vi "(SubVI)Serial_FGV.vi"(5 "Serial Settings (for init)":T2={"baud rate"=19200, "data bits"=8, "parity"=enum."None", "stop bits"=10, "flow control"=0} {"flow control" items=["None"=0, "XON/XOFF"=1, "RTS/CTS"=2, "DTR/DSR"=4]; "stop bits" items=["1.0"=10, "1.5"=15, "2.0"=20]; "data bits" min=5 max=8 step=1; "baud rate" items=["75"=75, "110"=110, "134"=134, "150"=150, "300"=300, "600"=600, "1200"=1200, "1800"=1800, "2400"=2400, "4800"=4800, "7200"=7200, "9600"=9600, "14400"=14400, "921600"=19200, "28800"=28800, "38400"=38400, "56000"=56000, "57600"=57600, "115200"=115200, "128000"=128000, "230400"=230400, "9216000"=921600, "1843200"=1843200]}, 7 "Function":T1=enum."Read", 8 "error in (no error)":errorcluster, 9 "Data to Write":string, 10 "Bytes to Read":u32, 11 "VISA resource name":refnum<visa-resource-name> caption="VISA In (for init)") -> (0 "error out":errorcluster, 2 "Read Data":string, 3 "VISA resource name out":refnum<visa-resource-name> caption="VISA Out")   [LabVIEW 2020]
uses:
  Controls/(Ctrl)Serial_FGV Function.ctl
  <vilib>/Instr/_visa.llb/VISA Flush IO Buffer Mask.ctl
  <vilib>/Instr/_visa.llb/VISA Configure Serial Port (Instr).vi
panel:
  in  "count":i32
  out "x-y":i32
  out "byte2":u32
  out "크기":i32
  out "byte":u32
  # "(SubVI)Serial_FGV.vi By hspark\n\nDescription : Serial 통신을 위한 기능적 글로벌 변수. 이 VI 안에서는 읽기, 쓰기 등 기본적인 기능만 수행해야 함\n\nInput : \n1. VISA In (for Init) : Initialize 시 Serial Port 설정을 위한 VISA 참조 입력\n2. Bytes to Read : Read 시 읽을 바이트 크기\n3. Data to Write : Write 시 Write 할 데이터 (String) \n4. Function : 초기화, 읽기, 쓰기 등 동작 입력\n5. Serial Setting (for Init) Initialize 시 Serial Port 설정을 위한 설정 값 입력 \n\nOutput : \n1. Read Data : Read 동작 시 읽은 데이터 (String)\n\nLabVIEW Version : 2020 SP1 이상\n\nNote : \n1. 시리얼 통신 오버런 에러 관련 테스트 필요 (0xBFFF006C)\n2. 시리얼 통신 디버깅 필요 시 케이스 구조 내 Serial Log 저장 코드 활성화 (모든 케이스에서 활성화해야 함)\n\nUpdate : 2021.11.03"
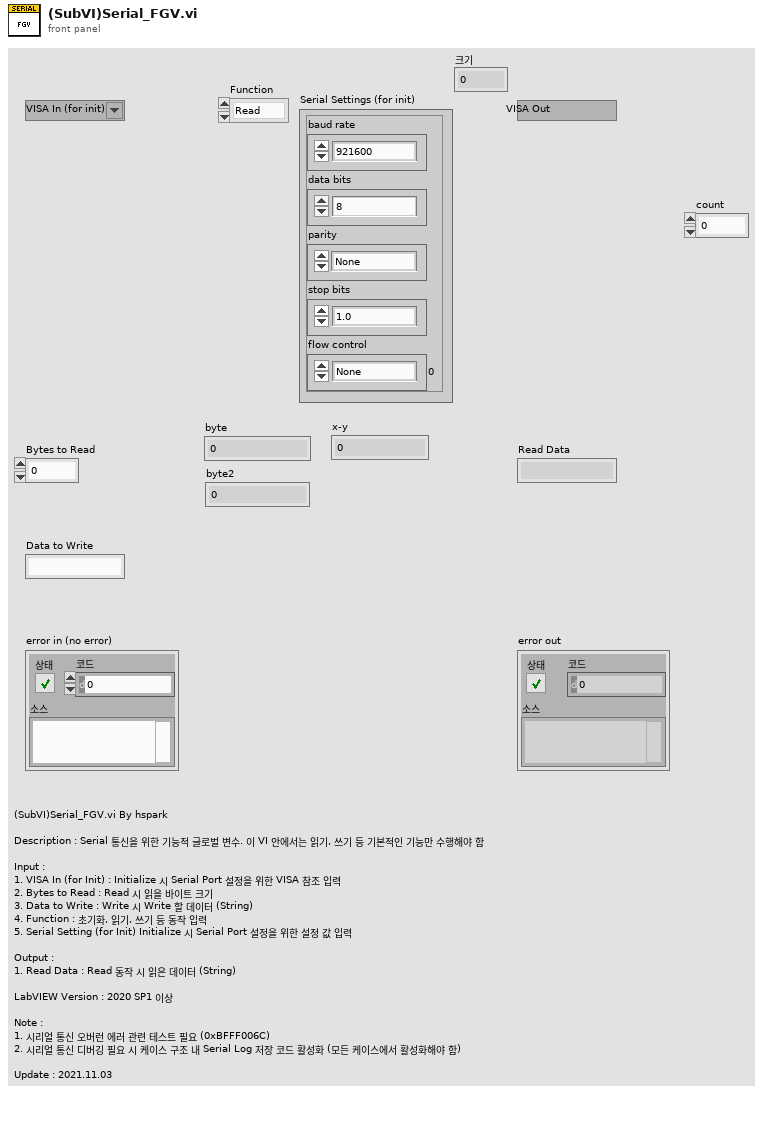
[diagram p1: front panel]
types:
  T1 = typedef "(Ctrl)Serial_FGV Function.ctl" = enum16{"Initialize", "Read", "Read All", "Write", "Flush Buffer", "Get Ref.", "Close"}
  T2 = cluster{"baud rate":u32, "data bits":u16, "parity":enum16{"None", "Odd", "Even", "Mark", "Space"}, "stop bits":u16, "flow control":u16}
  T3 = enum16{"open", "replace", "create", "open or create", "replace or create", "replace or create with confirmation"}
  T4 = typedef "VISA Flush IO Buffer Mask.ctl" = u16
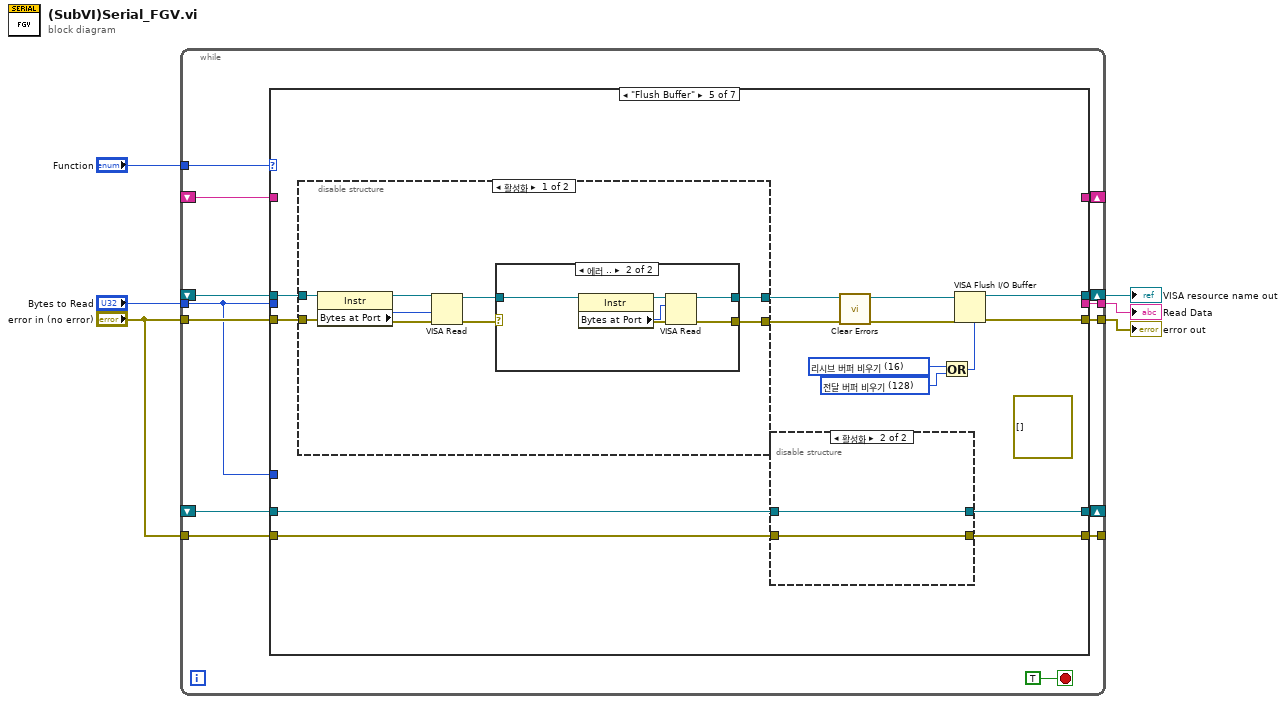
[diagram p0: block diagram]
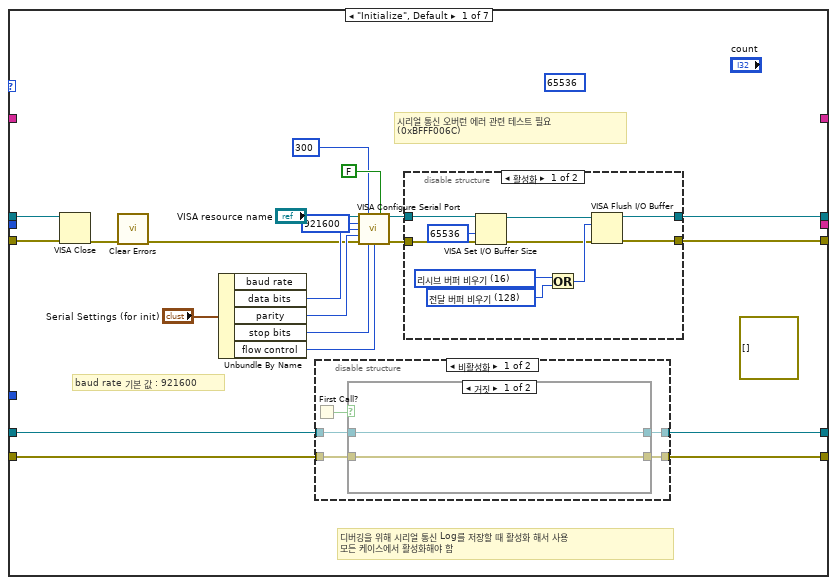
[diagram p2: hidden frame]
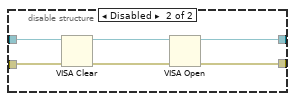
[diagram p3: hidden frame]
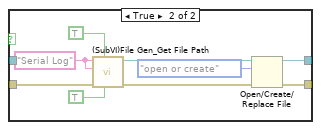
[diagram p4: hidden frame]
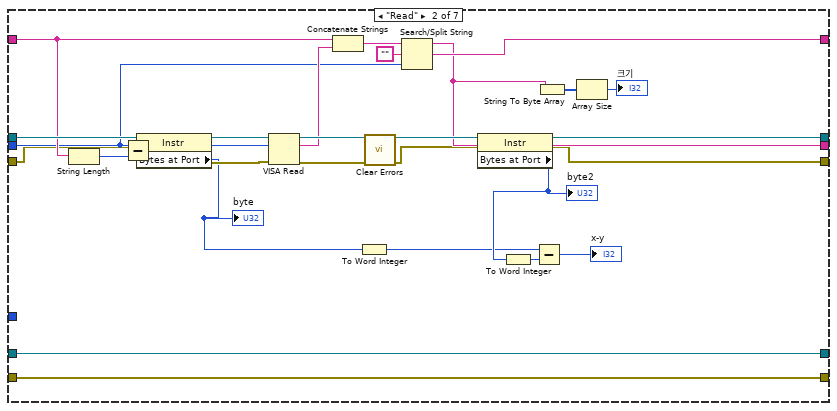
[diagram p6: hidden frame]
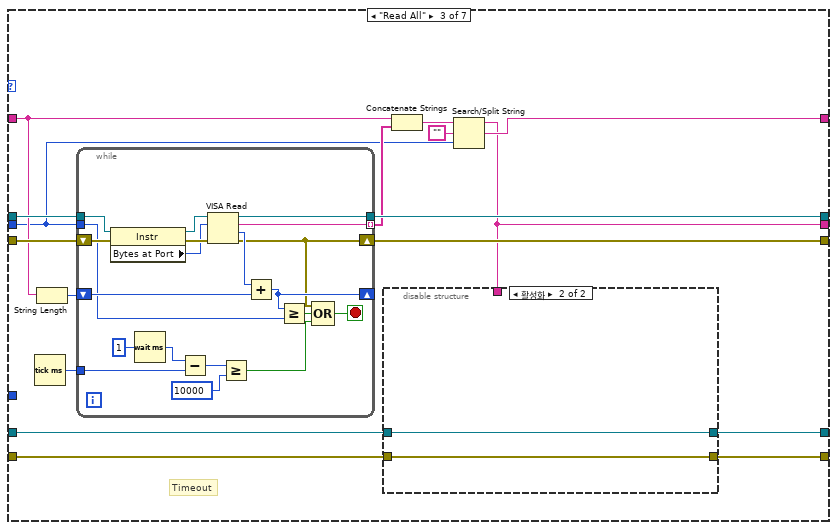
[diagram p7: hidden frame]
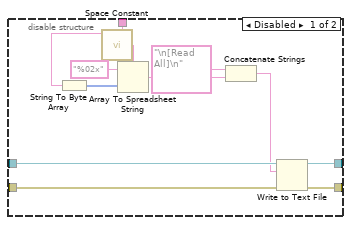
[diagram p8: hidden frame]
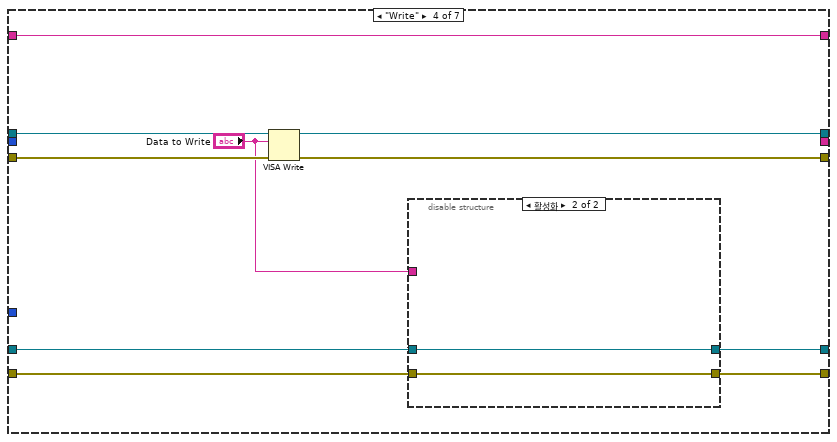
[diagram p9: hidden frame]
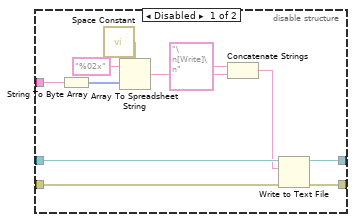
[diagram p10: hidden frame]
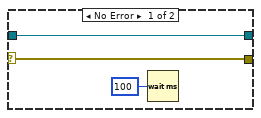
[diagram p11: hidden frame]
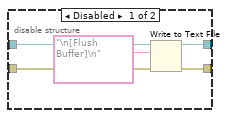
[diagram p13: hidden frame]
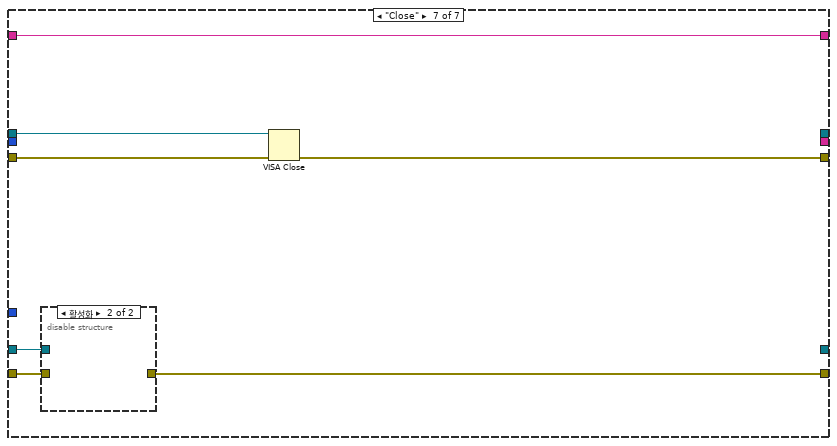
[diagram p15: hidden frame]
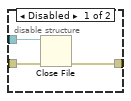
[diagram p16: hidden frame]
diagram:
  n1 = while {
    tunnel: "Function" -> [w18]
    shift-right: [w20] -> w6
    shift-left: _ -> [w17]
    tunnel: "error in (no error)" -> [w16]
    tunnel: [w15] -> w4
    shift-right: [w14] -> _
    shift-left: _ -> [w12]
    tunnel: [w13] -> _
    tunnel: "error in (no error)" -> [w11]
    shift-right: [w10] -> _
    shift-left: _ -> [w9]
    tunnel: "Bytes to Read" -> [w7]
    tunnel: [w8] -> w1
    stop <- TRUE stop-if-true
    n2 = case shown="\"Flush Buffer\"" w18 {
      tunnel: [w29 w84 w115 w157 w185 w215 _] -> w20
      tunnel: w17 -> [w24 w100 w114 w159 w187 w215 w224]
      tunnel: w16 -> [w27 w89 w117 w160 w177 w214 w225]
      tunnel: [w28 w81 w116 w158 w186 w214 w223] -> w15
      tunnel: [w34 w82 w110 w153 w179 w218 _] -> w14
      tunnel: [w33 w83 w111 w154 w180 w217 w220] -> w13
      tunnel: w12 -> [w23 w82 w113 w155 w178 w218 w221]
      tunnel: w11 -> [w32 w83 w112 w156 w181 w217 w222]
      tunnel: [_ w92 w106 w151 _ w216 w219] -> w10
      tunnel: w9 -> [_ w96 w104 w151 _ w216 w219]
      tunnel: w7 -> [_ w91 w102 _ _ _ _]
      tunnel: [_ w88 w105 _ _ _ _] -> w8
      tunnel: w7 -> [_ _ _ _ _ _ _]
      frame "Initialize", Default {
        (unwired) errorcluster[] [] ("배열")
        (unwired) u32 65536 ("크기(4096)")
        # "baud rate 기본 값 : 921600"
        # "디버깅을 위해 시리얼 통신 Log를 저장할 때 활성화 해서 사용\n모든 케이스에서 활성화해야 함"
        # "시리얼 통신 오버런 에러 관련 테스트 필요\n(0xBFFF006C)"
        n3 = VISA Close(VISA resource name=w24, error in (no error)=w27) -> (error out=w26:errorcluster)
        n4 = call <vilib>:"Clear Errors.vi"("error in (no error)"=w26) -> ("error out"=w25:errorcluster)  [unwired: 5 in, 1 out]
        n5 = Unbundle By Name("Serial Settings (for init)") -> ("data bits"=w39:u16, "parity"=w37:enum16{"None", "Odd", "Even", "Mark", "Space"}, "stop bits"=w40:u16, "flow control"=w41:u16)  [unwired: 1 out]
        n6 = disable-structure shown="비활성화" {
          disable-tunnel: [w62 _] -> w34
          disable-tunnel: [w61 _] -> w33
          disable-tunnel: w32 -> [w60 _]
          disable-tunnel: w23 -> [w58 _]
          frame Disabled {
            n7 = First Call?() -> (First Call?: T/F=w59:bool)
            n8 = case shown="거짓" w59 {
              tunnel: [w63 w73] -> w62
              tunnel: [w64 w72] -> w61
              tunnel: w60 -> [w64 w71]
              tunnel: w58 -> [w63 _]
              frame False {
              }
              frame True {
                w69 = "Serial Log" ("Folder Name")
                n9 = call "(SubVI)File Gen_Get File Path.vi"("Common?"=TRUE, "Use Timestamp"=TRUE, "error in (no error)"=w71, "File Name"=w69, "Folder Name"=w69) -> ("error out"=w67:errorcluster, "Path"=w68:path)  [unwired: 4 in, 1 out]
                n10 = Open/Create/Replace File(file path (use dialog)=w68, error in=w67, operation (0:open)=T3."open or create" ("동작(0:open)")) -> (refnum out=w73:refnum<file>, error out=w72:errorcluster)  [unwired: 3 in, 1 out]
              }
            }
          }
          frame Enabled {
          }
        }
        n11 = call-poly "VISA Configure Serial Port"("VISA resource name"="VISA resource name", "timeout (10sec)"=u32 300, "Enable Termination\nChar (T)"=FALSE ("Enable Termination\nChar (T)"), "baud rate (9600)"=u32 921600, "data bits (8)"=w39, "parity (0:none)"=w37, "error in (no error)"=w25, "stop bits (10: 1 bit)"=w40, "flow control (0:none)"=w41) -> ("VISA resource name out"=w31:refnum<visa-resource-name>, "error out"=w30:errorcluster)  [unwired: 5 out]
        n12 = disable-structure shown="활성화" {
          disable-tunnel: w31 -> [w48 w55]
          disable-tunnel: w30 -> [w47 w57]
          disable-tunnel: [w44 w52] -> w29
          disable-tunnel: [w43 w54] -> w28
          frame Enabled {
            w50 = T4 128 items=["리시브 버퍼 비우기"=16, "전달 버퍼 디바이스에 쓰기"=32, "리시브 버퍼 비우기(I/O 없음)"=64, "전달 버퍼 비우기"=128] ("Mask")
            w51 = T4 16 items=["리시브 버퍼 비우기"=16, "전달 버퍼 디바이스에 쓰기"=32, "리시브 버퍼 비우기(I/O 없음)"=64, "전달 버퍼 비우기"=128] ("Mask")
            n13 = VISA Set I/O Buffer Size(VISA resource name=w48, size (4096)=u32 65536 ("크기(4096)"), error in (no error)=w47) -> (VISA resource name out=w46:refnum<visa-resource-name>, error out=w45:errorcluster)  [unwired: 1 in]
            n14 = Or(x=w51, y=w50) -> (x .or. y?=w49:T4)
            n15 = VISA Flush I/O Buffer(VISA resource name=w46, mask (16)=w49, error in (no error)=w45) -> (VISA resource name out=w44:refnum<visa-resource-name>, error out=w43:errorcluster)
          }
          frame Disabled {
            n16 = VISA Clear(VISA resource name=w55, error in (no error)=w57) -> (VISA resource name out=w53:refnum<visa-resource-name>, error out=w56:errorcluster)
            n17 = VISA Open(error in (no error)=w56, VISA resource name=w53) -> (VISA resource name=w52:refnum<visa-resource-name>, error out=w54:errorcluster)  [unwired: 3 in]
          }
        }
      }
      frame "Read" {
        n18 = String Length(string=w96) -> (length=w97:i32)
        n19 = Subtract(x=w91, y=w97) -> (x-y=w93:u32)
        n20 = property class="Instr"(reference=w100, error in=w89) -> (reference out=w90:refnum<visa-resource-name>, error out=w85:errorcluster, "Bytes at Port"=w74:u32)
        "byte" <- w74
        n21 = VISA Read ("VISA 읽기")(VISA resource name=w90, byte count=w93, error in (no error)=w85) -> (VISA resource name out=w99:refnum<visa-resource-name>, read buffer=w98:string, error out=w77:errorcluster)  [unwired: 1 out]
        n22 = Concatenate Strings(w96, w98) -> (w94:string)
        n23 = To Word Integer(number=w74) -> (16bit integer=w76:i16)
        n24 = call <vilib>:"Clear Errors.vi"("error in (no error)"=w77) -> ("error out"=w78:errorcluster)  [unwired: 5 in, 1 out]
        n25 = Search/Split String(string=w94, search string/char (-)="", offset (0)=w91) -> (substring before match=w88:string, match + rest of string=w92:string)  [unwired: 1 out]
        n26 = property class="Instr"(reference=w99, error in=w78) -> (reference out=w84:refnum<visa-resource-name>, error out=w81:errorcluster, "Bytes at Port"=w80:u32)
        "byte2" <- w80
        n27 = To Word Integer(number=w80) -> (16bit integer=w75:i16)
        n28 = Subtract(x=w76, y=w75) -> (x-y=→"x-y":i16)
        n29 = String To Byte Array(string=w88) -> (unsigned byte array=w87:u8[])
        n30 = Array Size(array=w87) -> (size(s)=→"크기":i32)
      }
      frame "Read All" {
        # "Timeout"
        n31 = Tick Count (ms)() -> (millisecond timer value=w101:u32)
        n32 = String Length(string=w104) -> (length=w103:i32)
        n33 = while {
          tunnel: [w136] -> w115
          tunnel: w114 -> [w134]
          tunnel: [w132] -> w109 mode=indexing
          shift-right: [w125] -> w116
          shift-left: w117 -> [w137]
          shift-right: [w128] -> _
          shift-left: w103 -> [w131]
          tunnel: w102 -> [w127]
          tunnel: w101 -> [w122]
          stop <- w118 stop-if-true
          n34 = property class="Instr"(reference=w134, error in=w137) -> (reference out=w133:refnum<visa-resource-name>, error out=w135:errorcluster, "Bytes at Port"=w130:u32)
          n35 = Wait (ms)(milliseconds to wait=u32 1 ("대기 시간 (ms)")) -> (millisecond timer value=w123:u32)
          n36 = Subtract(x=w123, y=w122) -> (x-y=w121:u32)
          n37 = VISA Read ("VISA 읽기")(VISA resource name=w133, byte count=w130, error in (no error)=w135) -> (VISA resource name out=w136:refnum<visa-resource-name>, read buffer=w132:string, return count=w129:u32, error out=w125:errorcluster)
          n38 = Greater Or Equal?(x=w121, y=u32 10000) -> (x >= y?=w119:bool)
          n39 = Add(x=w129, y=w131) -> (x+y=w128:u32)
          n40 = Greater Or Equal?(x=w128, y=w127) -> (x >= y?=w126:bool)
          n41 = Compound Arithmetic op=OR(w125, w126, w119) -> (w118:bool)
        }
        n42 = Concatenate Strings(w104, w109) -> (w108:string)
        n43 = Search/Split String(string=w108, search string/char (-)="", offset (0)=w102) -> (substring before match=w105:string, match + rest of string=w106:string)  [unwired: 1 out]
        n44 = disable-structure shown="활성화" {
          disable-tunnel: w113 -> [w148 w150]
          disable-tunnel: w112 -> [w147 w149]
          disable-tunnel: [w146 w149] -> w111
          disable-tunnel: [w145 w150] -> w110
          disable-tunnel: w105 -> [w144 _]
          frame Disabled {
            n45 = String To Byte Array(string=w144) -> (unsigned byte array=w143:u8[])
            n46 = call <vilib>:"Space Constant.vi"() -> ("String"=w142:string)
            n47 = Array To Spreadsheet String(delimiter (Tab)=w142, array=w143, 3:"%02x" ("포맷 문자열")) -> (spreadsheet string=w141:string)
            n48 = Concatenate Strings("\n[Read All]\n" ("문자열"), w141) -> (w140:string)
            n49 = Write to Text File(file (use dialog)=w148, text=w140, error in=w147) -> (refnum out=w145:refnum<file>, error out=w146:errorcluster)  [unwired: 1 in, 1 out]
          }
          frame Enabled {
          }
        }
      }
      frame "Write" {
        n50 = VISA Write(VISA resource name=w159, write buffer="Data to Write", error in (no error)=w160) -> (VISA resource name out=w157:refnum<visa-resource-name>, error out=w158:errorcluster)  [unwired: 1 out]
        n51 = disable-structure shown="활성화" {
          disable-tunnel: w156 -> [w171 w172]
          disable-tunnel: w155 -> [w170 w173]
          disable-tunnel: [w169 w172] -> w154
          disable-tunnel: [w168 w173] -> w153
          disable-tunnel: "Data to Write" -> [w167 _]
          frame Disabled {
            n52 = String To Byte Array(string=w167) -> (unsigned byte array=w166:u8[])
            n53 = call <vilib>:"Space Constant.vi"() -> ("String"=w165:string)
            n54 = Array To Spreadsheet String(delimiter (Tab)=w165, array=w166, 3:"%02x" ("포맷 문자열")) -> (spreadsheet string=w164:string)
            n55 = Concatenate Strings("\n[Write]\n" ("문자열"), w164) -> (w163:string)
            n56 = Write to Text File(file (use dialog)=w170, text=w163, error in=w171) -> (refnum out=w168:refnum<file>, error out=w169:errorcluster)  [unwired: 1 in, 1 out]
          }
          frame Enabled {
          }
        }
      }
      frame "Flush Buffer" {
        (unwired) errorcluster[] [] ("배열")
        w184 = T4 128 items=["리시브 버퍼 비우기"=16, "전달 버퍼 디바이스에 쓰기"=32, "리시브 버퍼 비우기(I/O 없음)"=64, "전달 버퍼 비우기"=128] ("Mask")
        w183 = T4 16 items=["리시브 버퍼 비우기"=16, "전달 버퍼 디바이스에 쓰기"=32, "리시브 버퍼 비우기(I/O 없음)"=64, "전달 버퍼 비우기"=128] ("Mask")
        n57 = disable-structure shown="활성화" {
          disable-tunnel: w187 -> [w196 w206]
          disable-tunnel: w177 -> [w195 _]
          disable-tunnel: [w189 w206] -> w176
          disable-tunnel: [w188 _] -> w175
          frame Enabled {
            n58 = property class="Instr"(reference=w196, error in=w195) -> (reference out=w193:refnum<visa-resource-name>, error out=w194:errorcluster, "Bytes at Port"=w192:u32)
            n59 = VISA Read(VISA resource name=w193, byte count=w192, error in (no error)=w194) -> (VISA resource name out=w190:refnum<visa-resource-name>, error out=w191:errorcluster)  [unwired: 2 out]
            n60 = case shown="에러 .." w191 {
              selector: w191 -> [w198 _]
              tunnel: w190 -> [w199 w205]
              tunnel: [w199 w204] -> w189
              tunnel: [w198 w203] -> w188
              frame No Error {
                n61 = Wait (ms)(milliseconds to wait=u32 100 ("대기 시간 (ms)")) -> ()  [unwired: 1 out]
              }
              frame Error {
                n62 = property class="Instr"(reference=w205) -> (reference out=w202:refnum<visa-resource-name>, error out=w201:errorcluster, "Bytes at Port"=w200:u32)  [unwired: 1 in]
                n63 = VISA Read(VISA resource name=w202, byte count=w200, error in (no error)=w201) -> (VISA resource name out=w204:refnum<visa-resource-name>, error out=w203:errorcluster)  [unwired: 2 out]
              }
            }
          }
          frame Disabled {
          }
        }
        n64 = disable-structure shown="활성화" {
          disable-tunnel: w181 -> [w211 w212]
          disable-tunnel: [w210 w212] -> w180
          disable-tunnel: [w209 w213] -> w179
          disable-tunnel: w178 -> [w208 w213]
          frame Disabled {
            n65 = Write to Text File(file (use dialog)=w208, text="\n[Flush Buffer]\n" ("텍스트"), error in=w211) -> (refnum out=w209:refnum<file>, error out=w210:errorcluster)  [unwired: 1 in, 1 out]
          }
          frame Enabled {
          }
        }
        n66 = call <vilib>:"Clear Errors.vi"("error in (no error)"=w175) -> ("error out"=w174:errorcluster)  [unwired: 5 in, 1 out]
        n67 = Or(x=w183, y=w184) -> (x .or. y?=w182:T4)
        n68 = VISA Flush I/O Buffer(VISA resource name=w176, mask (16)=w182, error in (no error)=w174) -> (VISA resource name out=w185:refnum<visa-resource-name>, error out=w186:errorcluster)
      }
      frame "Get Ref." {
      }
      frame "Close" {
        n69 = disable-structure shown="활성화" {
          disable-tunnel: w222 -> [w228 _]
          disable-tunnel: w221 -> [w227 _]
          disable-tunnel: [w226 _] -> w220
          frame Disabled {
            n70 = Close File(refnum=w227, error in=w228) -> (error out=w226:errorcluster)  [unwired: 1 out]
          }
          frame Enabled {
          }
        }
        n71 = VISA Close(VISA resource name=w224, error in (no error)=w225) -> (error out=w223:errorcluster)
      }
    }
  }
  "VISA resource name out" <- w6
  "error out" <- w4
  "Read Data" <- w1
